vi "Set Duty Cycle.vi"(8 "Error In":errorcluster, 9 "Duty Cycles (0-255)":u8[](array[numeric]), 10 "Channels":u8[](array[numeric]), 11 "LINX Device Config":T1) -> (0 "Error Out":errorcluster, 3 "LINX Device Config":T1)   [LabVIEW 2020, in "Device.lvlib"]
doc: "Set the duty cycle of the specified PWM channels. A duty cylce of 0 is fully off while a duty cylce of 255 is fully on. A duty cycle of 127 is 50% on."
uses:
  Device.lvlib
  Type Defs/Error Type.ctl
  LMH-LINX.lvlib
  Type Defs/Interface.ctl
  Type Defs/Channels.ctl
  Type Defs/TCP Config.ctl
  Type Defs/LINX Device Config.ctl
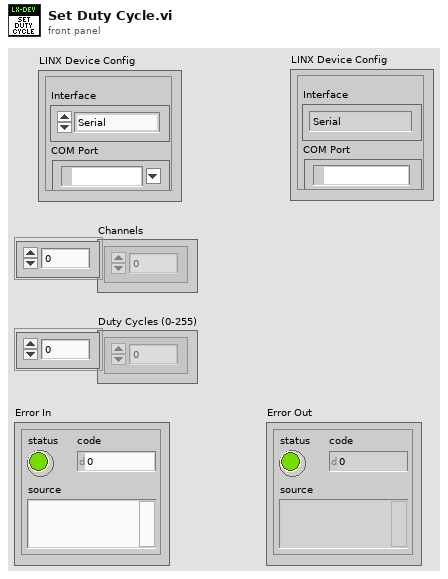
[diagram p1: front panel]
types:
  T1 = typedef "Device.lvlib/LINX Device Config.ctl" = cluster{"Interface":T2, "COM Port":refnum<visa-resource-name>, "TCP Configuration":T3, "Device Family":u8, "Device ID":u8, "Device Name":string, "TCP Ref":refnum<k5>, "Channels":T4}
  T2 = typedef "LMH-LINX.lvlib/Interface.ctl" = enum16{"Serial", "TCP"}
  T3 = typedef "Device.lvlib/TCP Config.ctl" = cluster{"IP Address":string, "Port":u16}
  T4 = typedef "LMH-LINX.lvlib/Channels.ctl" = cluster{"DI":u8[], "DO":u8[], "AI":u8[], "AO":u8[], "PWM":u8[], "QE":u8[], "UART":u8[], "I2C 2":u8[], "SPI":u8[], "CAN":u8[], "Servo":u8[], "AI Ref (V)":dbl, "AI Resolution (Bits)":u8, "AO Ref (V)":dbl, "AO Resolution (Bits)":u8}
  T5 = typedef "LMH-LINX.lvlib/Error Type.ctl" = enum16{"Unknown", "Timeout", "Corrupt Return Packet", "Unable To Connect", "Command Not Supported", "Channel DNE", "Invalid COM Config", "Firmware Version Mismatch", "myRIO Support", "CMD Specific Error", "Local IO Not Supported"}
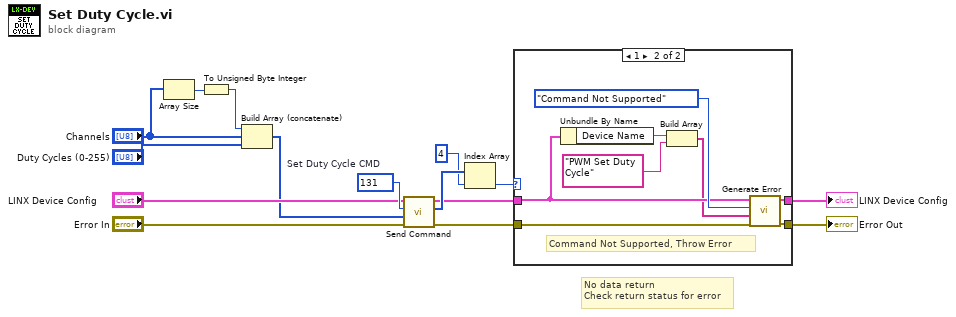
[diagram p0: block diagram]
diagram:
  w14 = u16 131  # Set Duty Cycle CMD
  # "No data return\nCheck return status for error"
  n1 = Array Size(array="Channels") -> (size(s)=w12:i32)
  n2 = To Unsigned Byte Integer(number=w12) -> (unsigned 8bit integer=w11:u8)
  n3 = Build Array (concatenate)(w11, "Channels", "Duty Cycles (0-255)") -> (w10:u8[])
  n4 = call "Send Command.vi"("Error In"="Error In", "ARGS"=w10, "CMD"=w14, "LINX Device Config"="LINX Device Config") -> ("Error Out"=w3:errorcluster, "Response"=w9:u8[], "LINX Device Config"=w5:T1)  [unwired: 4 in, 1 out]
  n5 = Index Array(array=w9, index=4) -> (element=w7:u8)
  n6 = case shown="1" w7 {
    tunnel: [w17 w23] -> w6
    tunnel: w5 -> [w17 w19]
    tunnel: [w16 w24] -> w4
    tunnel: w3 -> [w16 w25]
    frame 0, Default {
      # "Status OK"
    }
    frame 1 {
      # "Command Not Supported, Throw Error"
      n7 = Unbundle By Name(w19) -> ("Device Name"=w21:string)
      n8 = Build Array(w21, "PWM Set Duty Cycle") -> (w18:string[])
      n9 = call "Generate Error.vi"("Error In"=w25, "Arguments"=w18, "Error Type"=Error_Type."Command Not Supported", "LINX Device Config"=w19) -> ("Error Out"=w24:errorcluster, "Dup LINX Device Config"=w23:T1)  [unwired: 6 in]
    }
  }
  "Error Out" <- w4
  "LINX Device Config" <- w6
